vi "SSI PR or LD Pump Test.vi"() -> ()   [LabVIEW 2018, in "SSI PR or LD Pump.lvlib"]
uses:
  SSI PR or LD Pump.lvlib
  SSI PR or LD Settings Cluster.ctl
panel:
  out "Pressure":dbl format="%#_13g"
  in  "speed (ml/min)":dbl min=0.0 max=999.99 format="%06.2f"
  in  "?":bool
  out "Pump On?":enum16{"Off", "On", "Not Initialized"}(ring)
  out "Flow":dbl
  out "Connection Error":bool
  in  "Pause":bool
  out "Initialized":bool
  out "No Pump Connected":bool
  out "error out":errorcluster
  in  "error in (no error)":errorcluster
  out "SSI PR Settings Out":T1={"VISA resource name"="", "Simulated?"=TRUE}
  in  "SSI PR Settings In":T1
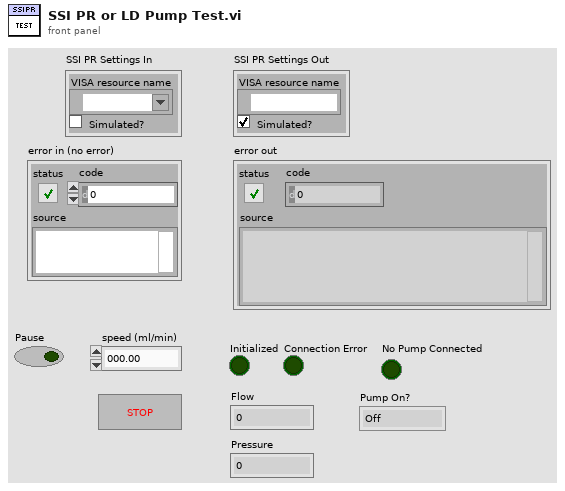
[diagram p1: front panel]
types:
  T1 = typedef "SSI PR or LD Pump.lvlib/SSI PR or LD Settings Cluster.ctl" = cluster{"VISA resource name":refnum<visa-resource-name>, "Simulated?":bool}
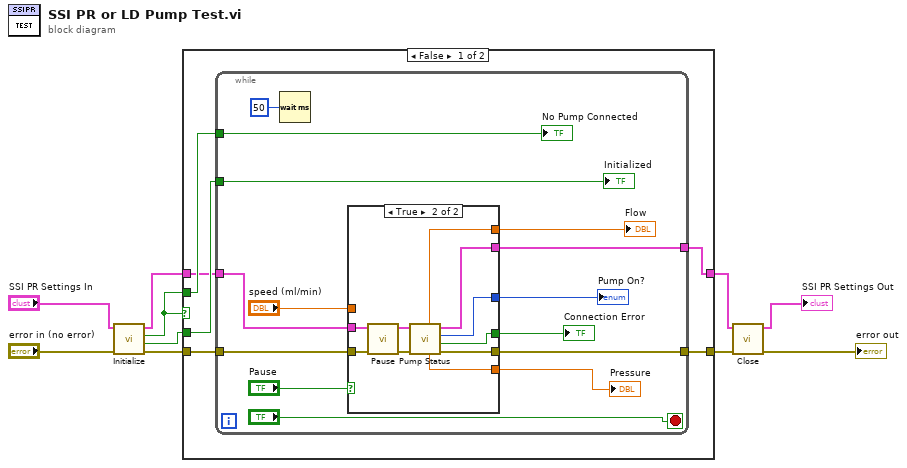
[diagram p0: block diagram]
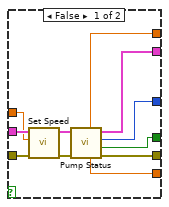
[diagram p2: hidden frame]
diagram:
  n1 = call "Initialize.vi"("error in (no error)"="error in (no error)", "SSI PR Settings In"="SSI PR Settings In") -> ("error out"=w2:errorcluster, "Initialized"=w6:bool, "No Pump Connected"=w1:bool, "SSI PR Settings Out"=w4:T1)  [unwired: 6 in]
  n2 = case shown="False" w1 {
    tunnel: w1 -> [w16 _]
    tunnel: w6 -> [w15 _]
    tunnel: [w14 w52] -> w5
    tunnel: w4 -> [w13 w52]
    tunnel: [w12 w53] -> w3
    tunnel: w2 -> [w11 w53]
    frame False {
      n3 = while {
        tunnel: w16 -> [w24]
        tunnel: w15 -> [w25]
        tunnel: [w30] -> w14
        tunnel: w13 -> [w29]
        tunnel: [w28] -> w12
        tunnel: w11 -> [w27]
        stop <- "?" stop-if-true
        n4 = Wait (ms)(milliseconds to wait=u32 50) -> ()  [unwired: 1 out]
        n5 = case shown="True" "Pause" {
          tunnel: [w37 w46] -> w30
          tunnel: w29 -> [w41 w51]
          tunnel: [w36 w47] -> w28
          tunnel: w27 -> [w40 w50]
          tunnel: [w35 w45] -> w22
          tunnel: [w32 w43] -> w21
          tunnel: [w34 w44] -> w23
          tunnel: "speed (ml/min)" -> [w33 _]
          tunnel: [w31 w42] -> w18
          frame False {
            n6 = call "Set Speed.vi"("error in (no error)"=w40, "speed (ml/min)"=w33, "SSI PR Settings In"=w41) -> ("error out"=w38:errorcluster, "SSI PR Settings Out"=w39:T1)  [unwired: 6 in, 1 out]
            n7 = call "Pump Status.vi"("error in (no error)"=w38, "SSI PR Settings"=w39) -> ("error out"=w36:errorcluster, "Connection Error"=w35:bool, "Pump On?"=w34:enum16{"Off", "On", "Not Initialized"}, "SSI PR Settings"=w37:T1, "Pressure"=w31:dbl, "Flow"=w32:dbl)  [unwired: 4 in]
          }
          frame True {
            n8 = call "Pause.vi"("error in (no error)"=w50, "SSI PR Settings In"=w51) -> ("error out"=w48:errorcluster, "SSI PR Settings Out"=w49:T1)  [unwired: 6 in, 1 out]
            n9 = call "Pump Status.vi"("error in (no error)"=w48, "SSI PR Settings"=w49) -> ("error out"=w47:errorcluster, "Connection Error"=w45:bool, "Pump On?"=w44:enum16{"Off", "On", "Not Initialized"}, "SSI PR Settings"=w46:T1, "Pressure"=w42:dbl, "Flow"=w43:dbl)  [unwired: 4 in]
          }
        }
        "Connection Error" <- w22
        "Pump On?" <- w23
        "Flow" <- w21
        "Pressure" <- w18
        "No Pump Connected" <- w24
        "Initialized" <- w25
      }
    }
    frame True {
    }
  }
  n10 = call "Close.vi"("error in (no error)"=w3, "SSI PR Settings In"=w5) -> ("error out"=→"error out":errorcluster, "SSI PR Settings Out"=→"SSI PR Settings Out":T1)  [unwired: 7 in, 1 out]
